vi "Sound Spectrum Example.vi"() -> ()   [LabVIEW 2016]
doc: "This VI illustrates how to perform simultaneous sound IO, i.e., how to continuously play the sound acquired from a microphone. It requires the use of a microphone attached to the sound card. You can specify the IDs of the input and output devices, the frequency to sample at, and the buffer size for both devices. Higher frequencies have better quality, but demand more resources and are limited by the capabilities of your sound card. A large number of samples decreases the risk of glitches, but increases the delay between acquisition and playback."
uses:
  <vilib>/Analysis/4window.llb/windowTd.ctl
  <vilib>/sound2/lvsound2.llb/Sampling Mode.ctl
  <vilib>/measure/maspectr.llb/Power Spectrum and PSD Export Mode.ctl
  <vilib>/sound2/lvsound2.llb/Sound Input Read (DBL).vi
  <vilib>/measure/maspectr.llb/FFT Power Spectrum and PSD for N Chan.vi
  <vilib>/measure/NI_MAPro.lvlib
  <vilib>/Analysis/NI_AALPro.lvlib
panel:
  in  "Tab Control":enum32{"Signal", "Settings"}(tab)
  out "Acquired Sound":waveform(dbl)[](graph)=[{"t0"=timestamp(3602439436.041315 s since 1904-01-01), "dt"=2.2675736961451248e-05, "Y"=array[8820 elements]}, {"t0"=timestamp(3602439436.041315 s since 1904-01-01), "dt"=2.2675736961451248e-05, "Y"=array[8820 elements]}]
  out "Power Spectral Density":cluster{"f0":dbl, "df":dbl, "magnitude":dbl[]}[](graph)=[{"f0"=0.0, "df"=5.0, "magnitude"=array[4410 elements]}, {"f0"=0.0, "df"=5.0, "magnitude"=array[4410 elements]}]
  in  "Sampling":T1={"Rate [S/s]"=44100.0, "Channels"=2.0, "Resolution [Bits]"=16.0} {"Rate [S/s]" format="%#_6p"}
  in  "Block Size [s]":dbl=0.2 min=0.1 max=5.0 step=0.1
  in  "Window":T2=1 items=["Rectangle"=0, "Hanning"=1, "Hamming"=2, "Blackman-Harris"=3, "Exact Blackman"=4, "Blackman"=5, "Flat Top"=6, "4 Term B-Harris "=7, "7 Term B-Harris"=8, "Low Sidelobe"=9, "Blackman Nuttall"=11, "Triangle"=30, "Bartlett-Hanning"=31, "Bohman"=32, "Parzen"=33, "Welch"=34, "Kaiser"=60, "Dolph-Chebyshev"=61, "Gaussian"=62]
  in  "Sound Input Device ID":u32
  in  "Stop":bool
  # "Sound Signal and Frequency Spectrum"
  # "Record sound from the computer input device.\nPlot the recorded signal in the time domain, and its power spectrum."
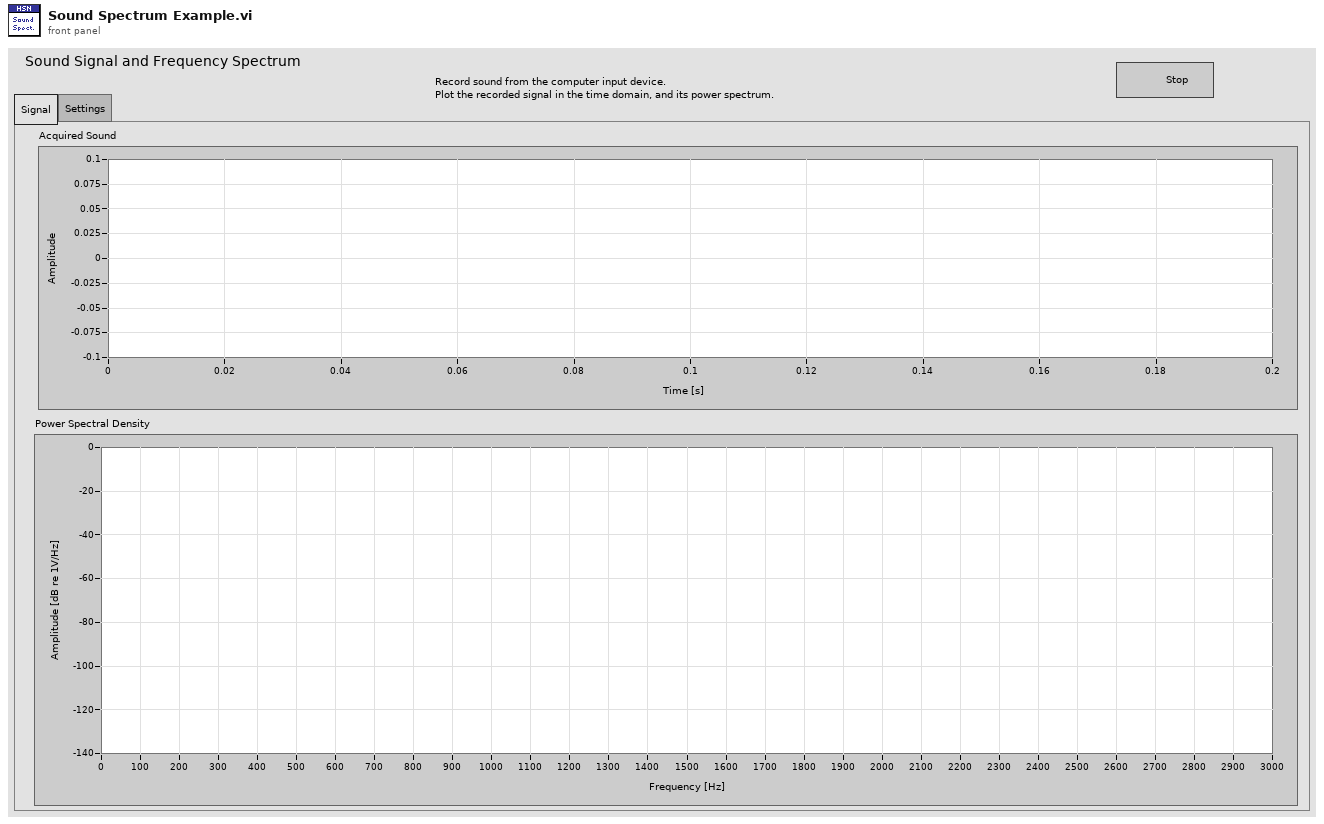
[diagram p1: front panel]
types:
  T1 = cluster{"Rate [S/s]":dbl, "Channels":dbl, "Resolution [Bits]":dbl}
  T2 = typedef "NI_AALPro.lvlib/windowTd.ctl" = u32
  T3 = typedef "Sampling Mode.ctl" = i32
  T4 = typedef "Sound Input Task ID.ctl" = u32
  T5 = typedef "NI_MAPro.lvlib/Power Spectrum and PSD Export Mode.ctl" = u16
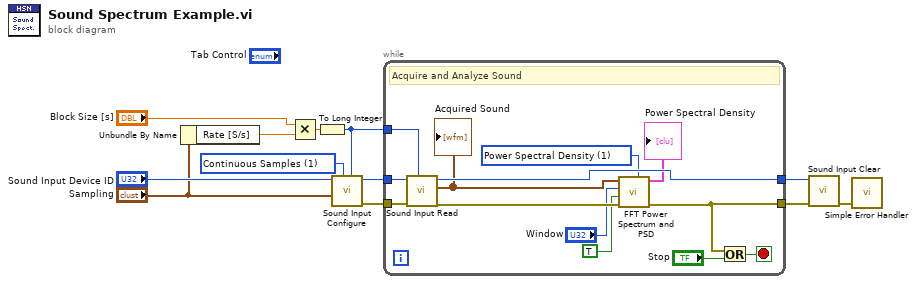
[diagram p0: block diagram]
diagram:
  w7 = T3 1 items=["Finite Samples", "Continuous Samples"] ("sample mode")
  n1 = Unbundle By Name("Sampling") -> ("Rate [S/s]"=w4:dbl)
  n2 = Multiply(x="Block Size [s]", y=w4) -> (x*y=w2:dbl)
  n3 = To Long Integer(number=w2) -> (32bit integer=w1:i32)
  n4 = call <vilib>:"Sound Input Configure.vi"("number of samples/ch"=w1, "sample mode"=w7, "sound format"="Sampling", "device ID"="Sound Input Device ID") -> ("error out"=w9:errorcluster, "task ID"=w8:T4)  [unwired: 6 in]
  n5 = while {
    tunnel: w1 -> [w23]
    tunnel: w8 -> [w24]
    tunnel: [w22] -> w10
    tunnel: w9 -> [w25]
    tunnel: [w18] -> w12
    stop <- w20 stop-if-true
    w14 = T5 1 items=["Power Spectrum", "Power Spectral Density"] ("export mode")
    # "Acquire and Analyze Sound"
    n6 = call-poly <vilib>:"Sound Input Read.vi"("number of samples/ch"=w23, "error in (no error)"=w25, "task ID"=w24) -> ("error out"=w17:errorcluster, "data"=w19:waveform(dbl)[], "task ID out"=w22:T4)  [unwired: 6 in]
    "Acquired Sound" <- w19
    n7 = call-poly <vilib>:"FFT Power Spectrum and PSD.vi"("export mode"=w14, "error in (no error)"=w17, "dB On (F)"=TRUE, "window"="Window", "time signals"=w19) -> ("error out"=w18:errorcluster, "Power Spectrum / PSD"=→"Power Spectral Density":cluster{"f0":dbl, "df":dbl, "magnitude":dbl[]}[])  [unwired: 3 in, 2 out]
    n8 = Or(x=w18, y="Stop") -> (x .or. y?=w20:bool)
  }
  n9 = call <vilib>:"Sound Input Clear.vi"("error in (no error)"=w12, "task ID"=w10) -> ("error out"=w6:errorcluster)  [unwired: 9 in]
  n10 = call <vilib>:"Simple Error Handler.vi"("error in (no error)"=w6) -> ()  [unwired: 4 in, 5 out]
